vi "Configure Pulse Mode.vi"(6 "channel":i32=1 min=1 max=4, 8 "error in (no error)":errorcluster, 10 "Pulse Mode (0: single)":T1 items=["Single", "Double", "Triple", "Quadruple", "External Width"], 11 "VISA resource name":refnum<visa-resource-name>) -> (0 "error out":errorcluster, 3 "VISA resource name out":refnum<visa-resource-name>)   [LabVIEW 2019, in "Pulse Rider PG-1000.lvlib"]
doc: "Sets the pulse mode for the selected output channel. It sets how many pulses will be available for the selected output; if 'external width' is selected it means that the Trigger In signal is directly routed to the selected output.\n\nchannel: the output channel int from 1 to 4\nmode: an available mode : 'external width', 'quadruple', 'triple', 'double', 'single'"
uses:
  <instrlib>/LV_PulseRiderPG1000/Pulse Rider PG-1000.lvlib
  <instrlib>/LV_PulseRiderPG1000/Public/Configure/Pulse/Pulse Mode.ctl
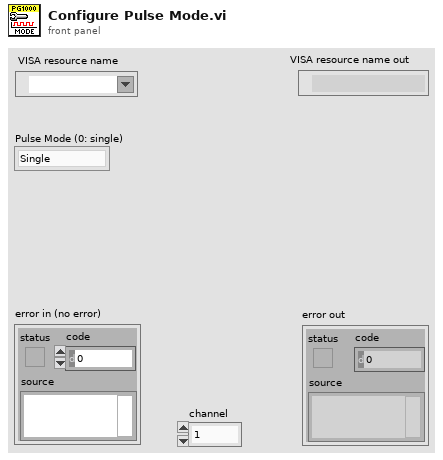
[diagram p1: front panel]
types:
  T1 = typedef "Pulse Rider PG-1000.lvlib/Pulse Mode.ctl" = u16
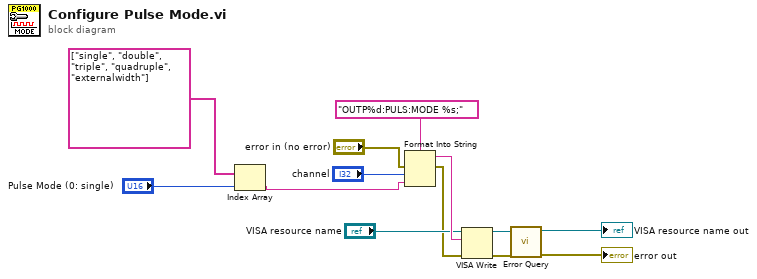
[diagram p0: block diagram]
diagram:
  n1 = Index Array(array=string[] ["single", "double", "triple", "quadruple", "externalwidth"], index="Pulse Mode (0: single)") -> (element=w3:string)
  n2 = Format Into String(format string="OUTP%d:PULS:MODE %s;", error in="error in (no error)", "channel", w3) -> (resulting string=w10:string, error out=w2:errorcluster)  [unwired: 1 in]
  n3 = VISA Write(VISA resource name="VISA resource name", write buffer=w10, error in (no error)=w2) -> (VISA resource name out=w13:refnum<visa-resource-name>, error out=w12:errorcluster)  [unwired: 1 out]
  n4 = call <instrlib>:"Error Query.vi"("error in (no error)"=w12, "VISA resource name"=w13) -> ("error out"=→"error out":errorcluster, "VISA resource name out"=→"VISA resource name out":refnum<visa-resource-name>)  [unwired: 6 in, 2 out]
